vi "calcolo delta t.vi"(6 "Tamb freddo":dbl, 8 "error out":errorcluster, 9 "Tamb":dbl, 10 "R freddo":dbl, 11 "R misurata":dbl) -> (0 "error out 2":errorcluster, 3 "Dt":dbl)   [LabVIEW 2019]
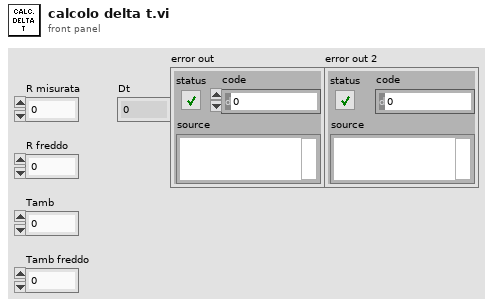
[diagram p1: front panel]
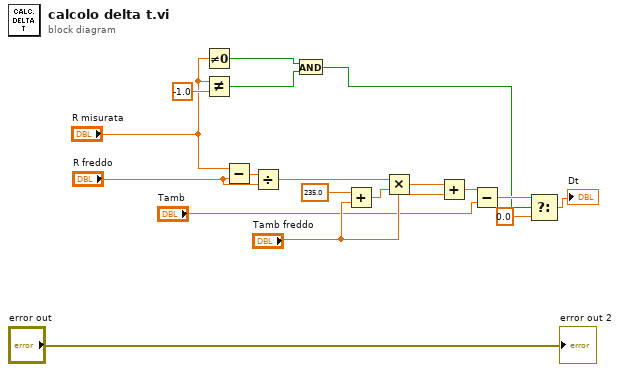
[diagram p0: block diagram]
diagram:
  n1 = Not Equal To 0?(x="R misurata") -> (x != 0?=w3:bool)
  n2 = Not Equal?(x="R misurata", y=-1.0) -> (x != y?=w2:bool)
  n3 = Subtract(x="R misurata", y="R freddo") -> (x-y=w10:dbl)
  n4 = Divide(x=w10, y="R freddo") -> (x/y=w11:dbl)
  n5 = And(x=w3, y=w2) -> (x .and. y?=w1:bool)
  n6 = Add(x=235.0, y="Tamb freddo") -> (x+y=w13:dbl)
  n7 = Multiply(x=w11, y=w13) -> (x*y=w14:dbl)
  n8 = Add(x=w14, y="Tamb freddo") -> (x+y=w15:dbl)
  n9 = Subtract(x=w15, y="Tamb") -> (x-y=w8:dbl)
  n10 = Select(t=w8, s=w1, f=0.0) -> (s? t:f=→"Dt":dbl)
  "error out 2" <- "error out"
